vi "Example.vi"() -> ()   [LabVIEW 2014]
uses:
  EventLogger_Actor Messages/LogsStringRef Msg/LogsStringRef Msg.lvclass/LogsStringRef Msg.ctl
  <vilib>/ActorFramework/Message Enqueuer/Message Enqueuer.lvclass/Message Enqueuer.ctl
  EventLogger_Actor Messages/ErrorBooleanRef Msg/ErrorBooleanRef Msg.lvclass/ErrorBooleanRef Msg.ctl
  EventLogger_Actor Messages/LogEvent Msg/LogEvent Msg.lvclass/LogEvent Msg.ctl
  EventLogger_Actor Messages/LogError Msg/LogError Msg.lvclass/LogError Msg.ctl
  <vilib>/ActorFramework/Message Enqueuer/Enqueue.vi
  <vilib>/ActorFramework/Message Priority Queue/Priority Enqueue.vi
  EventLogger_Actor Messages/LogsStringRef Msg/LogsStringRef Msg.lvclass
  EventLogger_Actor Messages/ErrorBooleanRef Msg/ErrorBooleanRef Msg.lvclass
  EventLogger_Actor Messages/LogEvent Msg/LogEvent Msg.lvclass
  EventLogger_Actor Messages/LogError Msg/LogError Msg.lvclass
  <vilib>/ActorFramework/Stop Msg/Stop Msg.lvclass
  EventLogger_Actor/EventLogger_Actor.lvclass
panel:
  out "Error?":bool
  out "String":string
  # "BSD 2-Clause License\n\nCopyright (c) 2018, Ajay www.digiajay.com\nAll rights reserved.\n\nRedistribution and use in source and binary forms, with or without\nmodification, are permitted provided that the following conditions are met:\n\n* Redistributions of source code must retain the above copyright notice, this\n  list of conditions and the following disclaimer.\n\n* Redistributions in binary form must reproduce the above copyright notice,\n  this list of conditions and the following disclaimer in the documentation\n  and/or other materials provided with the distribution.\n\nTHIS SOFTWARE IS PROVIDED BY THE COPYRIGHT HOLDERS AND CONTRIBUTORS \"AS IS\"\nAND ANY EXPRESS OR IMPLIED WARRANTIES, INCLUDING, BUT NOT LIMITED TO, THE\nIMPLIED WARRANTIES OF MERCHANTABILITY AND FITNESS FOR A PARTICULAR PURPOSE ARE\nDISCLAIMED. IN NO EVENT SHALL THE COPYRIGHT HOLDER OR CONTRIBUTORS BE LIABLE\nFOR ANY DIRECT, INDIRECT, INCIDENTAL, SPECIAL, EXEMPLARY, OR CONSEQUENTIAL\nDAMAGES (INCLUDING, BUT NOT LIMITED TO, PROCUREMENT OF SUBSTITUTE GOODS OR\nSERVICES; LOSS OF USE, DATA, OR PROFITS; OR BUSINESS INTERRUPTION) HOWEVER\nCAUSED AND ON ANY THEORY OF LIABILITY, WHETHER IN CONTRACT, STRICT LIABILITY,\nOR TORT (INCLUDING NEGLIGENCE OR OTHERWISE) ARISING IN ANY WAY OUT OF THE USE\nOF THIS SOFTWARE, EVEN IF ADVISED OF THE POSSIBILITY OF SUCH DAMAGE."
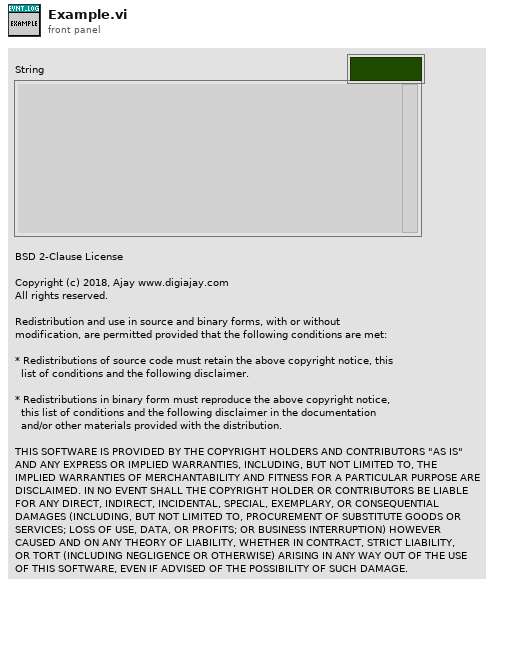
[diagram p1: front panel]
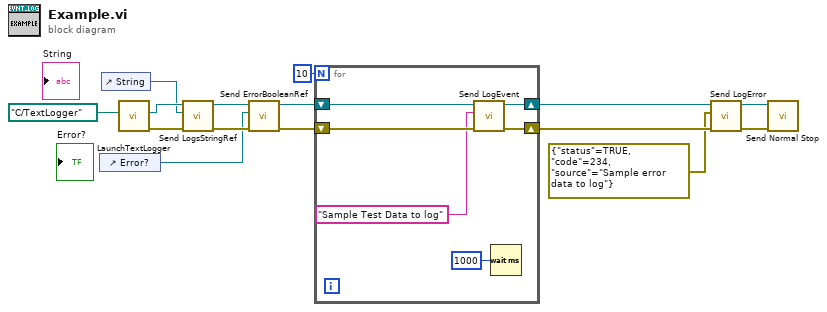
[diagram p0: block diagram]
diagram:
  n1 = control-ref of="Error?"() -> (w6:refnum<vi>)
  n2 = control-ref of="String"() -> (w10:refnum<vi>)
  n3 = call "LaunchTextLogger.vi"("Text Log Folder"=path "C:/TextLogger") -> ("error out"=w15:errorcluster, "Text Logger Actor's Enqueuer"=w11:refnum<class "Message Enqueuer.lvclass">)  [unwired: 8 in, 1 out]
  n4 = call "Send LogsStringRef.vi"("error in (no error)"=w15, "LogIndicatorStringRef"=w10, "Message Enqueuer"=w11) -> ("error out"=w12:errorcluster, "Message Enqueuer out"=w8:refnum<class "Message Enqueuer.lvclass">)  [unwired: 7 in]
  n5 = call "Send ErrorBooleanRef.vi"("error in (no error)"=w12, "Error Indicator Boolean Ref"=w6, "Message Enqueuer"=w8) -> ("error out"=w9:errorcluster, "Message Enqueuer out"=w7:refnum<class "Message Enqueuer.lvclass">)  [unwired: 7 in]
  n6 = for {
    N: 10 -> [_]
    shift-right: [w17] -> w2
    shift-left: w9 -> [w21]
    shift-right: [w20] -> w4
    shift-left: w7 -> [w19]
    n7 = call "Send LogEvent.vi"("error in (no error)"=w21, "Text Message to Log"="Sample Test Data to log", "Message Enqueuer"=w19) -> ("error out"=w17:errorcluster, "Message Enqueuer out"=w20:refnum<class "Message Enqueuer.lvclass">)  [unwired: 7 in]
    n8 = Wait (ms)(milliseconds to wait=u32 1000) -> ()  [unwired: 1 out]
  }
  n9 = call "Send LogError.vi"("error in (no error)"=w2, "ErrorToLog"=errorcluster {"status"=TRUE, "code"=234, "source"="Sample error data to log"}, "Message Enqueuer"=w4) -> ("error out"=w5:errorcluster, "Message Enqueuer out"=w3:refnum<class "Message Enqueuer.lvclass">)  [unwired: 7 in]
  n10 = call <vilib>:"Send Normal Stop.vi"("error in (no error)"=w5, "Message Enqueuer"=w3) -> ()  [unwired: 9 in, 1 out]
